vi "MoveSlideLocation.vi"(0 "old Table":string[][](table), 1 "start location":cluster{i32, i32}, 2 "end location":cluster{i32, i32}, 3 "name":string, 4 "order #":i32, 7 "Mod":T1=enum."Bounce") -> (5 "new Table":string[][](table), 6 "iterator":i32)   [LabVIEW 2012]
uses:
  SlideParams.ctl
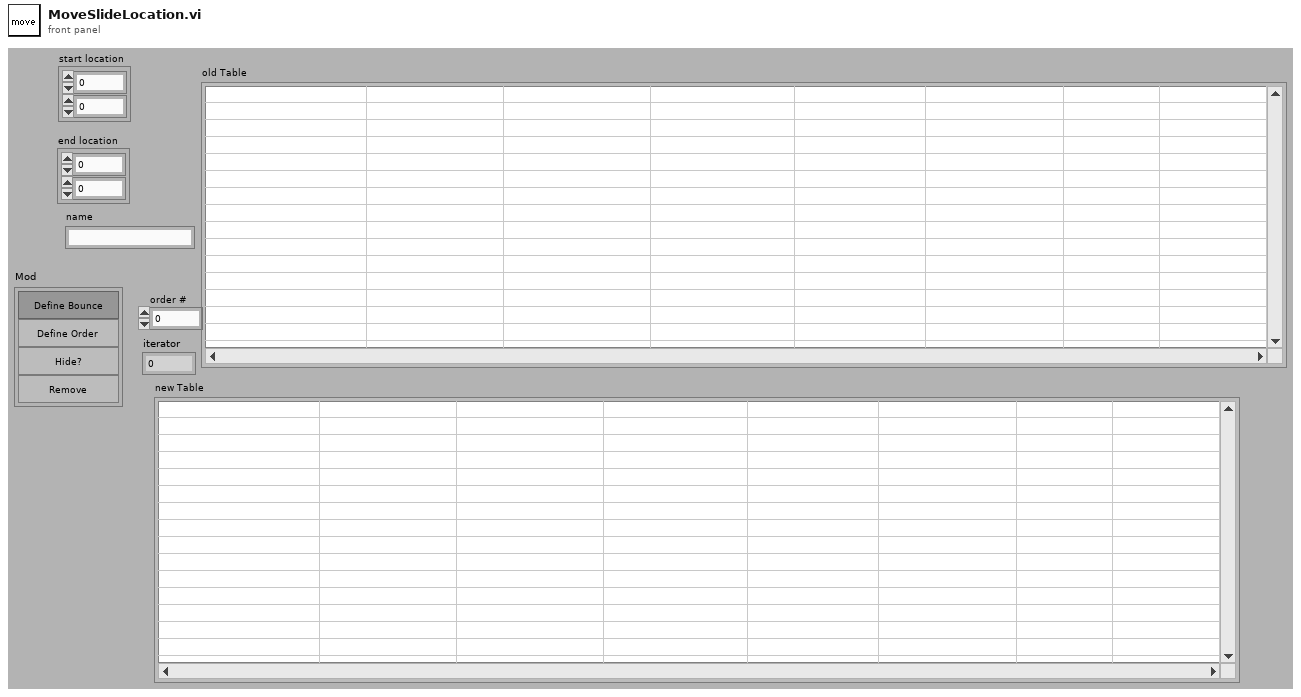
[diagram p1: front panel]
types:
  T1 = typedef "SlideParams.ctl" = enum32{"No Selection", "Bounce", "Order", "Hide", "Remove"}
  T2 = typedef "ParamterCluster.ctl" = cluster{"bounce?":bool, "black?":bool, "slide number":i32, "hide?":bool, "selection":bool}
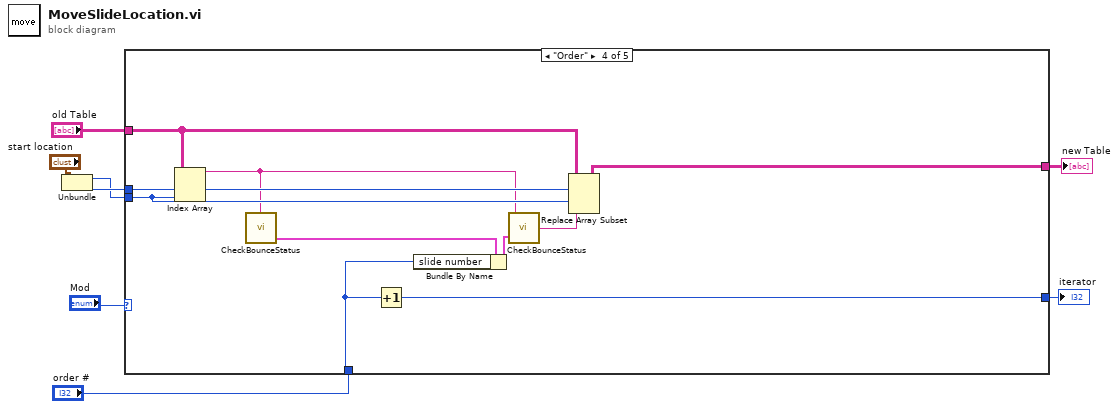
[diagram p0: block diagram]
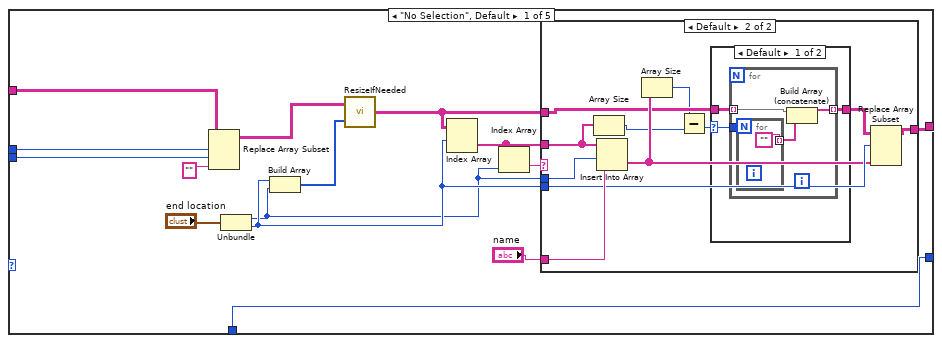
[diagram p2: hidden frame]
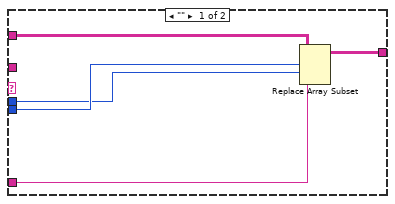
[diagram p3: hidden frame]
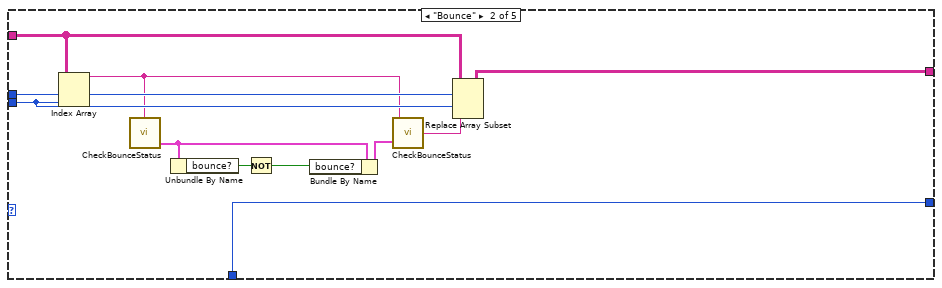
[diagram p5: hidden frame]
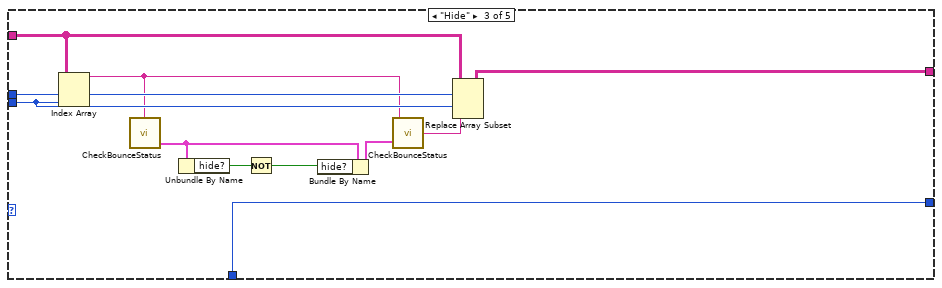
[diagram p6: hidden frame]
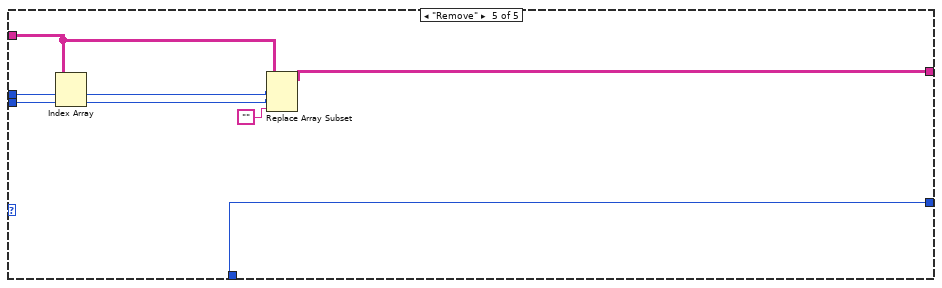
[diagram p7: hidden frame]
diagram:
  n1 = Unbundle("start location") -> (w6:i32, w7:i32)
  n2 = case shown="\"Order\"" "Mod" {
    tunnel: w7 -> [w15 w59 w70 w80 w85]
    tunnel: w6 -> [w14 w57 w68 w78 w84]
    tunnel: [w12 w56 w67 w77 w81] -> w5
    tunnel: "old Table" -> [w11 w58 w69 w79 w82]
    tunnel: "order #" -> [w9 w49 w60 w72 w86]
    tunnel: [w9 w49 w60 w71 w86] -> w2
    frame "No Selection", Default {
      n3 = Replace Array Subset(array=w11, new element="" ("name"), index (row)=w15, index (col)=w14) -> (w10:string[][])
      n4 = Unbundle("end location") -> (w18:i32, w19:i32)
      n5 = Build Array(w19, w18) -> (w17:i32[])
      n6 = call "ResizeIfNeeded.vi"("Size"=w17, "Table"=w10) -> ("Table out"=w16:string[][])
      n7 = Index Array(array=w16, index (row)=w19) -> (element=w20:string[])  [unwired: 1 in]
      n8 = Index Array(array=w20, index=w18) -> (element=w22:string)
      n9 = case shown="Default" w22 {
        tunnel: w16 -> [w28 w32]
        tunnel: w19 -> [w27 w37]
        tunnel: w18 -> [w26 w38]
        tunnel: "name" -> [w25 w39]
        tunnel: [w24 w36] -> w12
        tunnel: w20 -> [_ w35]
        frame "" {
          n10 = Replace Array Subset(array=w28, new element=w25, index (row)=w27, index (col)=w26) -> (w24:string[][])
        }
        frame Default {
          n11 = Array Size(array=w35) -> (size(s)=w30:i32)
          n12 = Insert Into Array(array=w35, index=w38, new element=w39) -> (w34:string[])
          n13 = Array Size(array=w34) -> (size(s)=w31:i32)
          n14 = Subtract(x=w31, y=w30) -> (x-y=w29:i32)
          n15 = case shown="Default" w29 {
            selector: w29 -> [w40 _]
            tunnel: [w41 w48] -> w33
            tunnel: w32 -> [w42 w48]
            frame Default {
              n16 = for {
                tunnel: w42 -> [w46] mode=indexing
                tunnel: [w45] -> w41 mode=indexing
                tunnel: w40 -> [w43]
                n17 = for {
                  N: w43 -> [_]
                  tunnel: [""] -> w44 mode=indexing
                }
                n18 = Build Array (concatenate)(w46, w44) -> (w45:string[])
              }
            }
            frame 0 {
            }
          }
          n19 = Replace Array Subset(array=w33, new element=w34, index (row)=w37) -> (w36:string[][])  [unwired: 1 in]
        }
      }
    }
    frame "Bounce" {
      n20 = Index Array(array=w58, index (row)=w59, index (col)=w57) -> (element=w54:string)
      n21 = call "CheckBounceStatus.vi"("File Name"=w54) -> ("Parameters"=w52:T2)  [unwired: 1 in, 2 out]
      n22 = Unbundle By Name(w52) -> ("bounce?"=w55:bool)
      n23 = Not(x=w55) -> (.not. x?=w53:bool)
      n24 = Bundle By Name(cluster=w52, "bounce?"=w53) -> (w51:T2)
      n25 = call "CheckBounceStatus.vi"("Parameters in"=w51, "File Name"=w54) -> ("With parameters"=w50:string)  [unwired: 2 out]
      n26 = Replace Array Subset(array=w58, new element=w50, index (row)=w59, index (col)=w57) -> (w56:string[][])
    }
    frame "Hide" {
      n27 = Index Array(array=w69, index (row)=w70, index (col)=w68) -> (element=w65:string)
      n28 = call "CheckBounceStatus.vi"("File Name"=w65) -> ("Parameters"=w63:T2)  [unwired: 1 in, 2 out]
      n29 = Unbundle By Name(w63) -> ("hide?"=w66:bool)
      n30 = Not(x=w66) -> (.not. x?=w64:bool)
      n31 = Bundle By Name(cluster=w63, "hide?"=w64) -> (w62:T2)
      n32 = call "CheckBounceStatus.vi"("Parameters in"=w62, "File Name"=w65) -> ("With parameters"=w61:string)  [unwired: 2 out]
      n33 = Replace Array Subset(array=w69, new element=w61, index (row)=w70, index (col)=w68) -> (w67:string[][])
    }
    frame "Order" {
      n34 = Index Array(array=w79, index (row)=w80, index (col)=w78) -> (element=w76:string)
      n35 = call "CheckBounceStatus.vi"("File Name"=w76) -> ("Parameters"=w75:T2)  [unwired: 1 in, 2 out]
      n36 = Increment(x=w72) -> (x+1=w71:i32)
      n37 = Bundle By Name(cluster=w75, "slide number"=w72) -> (w74:T2)
      n38 = call "CheckBounceStatus.vi"("Parameters in"=w74, "File Name"=w76) -> ("With parameters"=w73:string)  [unwired: 2 out]
      n39 = Replace Array Subset(array=w79, new element=w73, index (row)=w80, index (col)=w78) -> (w77:string[][])
    }
    frame "Remove" {
      n40 = Index Array(array=w82, index (row)=w85, index (col)=w84) -> ()  [unwired: 1 out]
      n41 = Replace Array Subset(array=w82, new element="", index (row)=w85, index (col)=w84) -> (w81:string[][])
    }
  }
  "new Table" <- w5
  "iterator" <- w2
